vi "生成与显示信号.vi"() -> ()   [LabVIEW 2010]
doc: "Use this template to generate a signal and display the generated data in a graph. \n\nUse this template with the exercises in the Getting Started with LabVIEW manual.\n\nNote: VIs created from this template will have automatic error handling enabled by default."
uses:
  Instance           1 22Saved   生成与显示信号 .vi
  Instance           2 22Saved   生成与显示信号 .vi
panel:
  out "最小值":dbl
  out "最大值":dbl
  out "算术平均值":dbl
  in  "噪声幅度":dbl(slide) scale=0.0..10.0
  out "Waveform Graph":dynamicdata(graph)
  in  "stop":bool
  # "生成与显示信号"
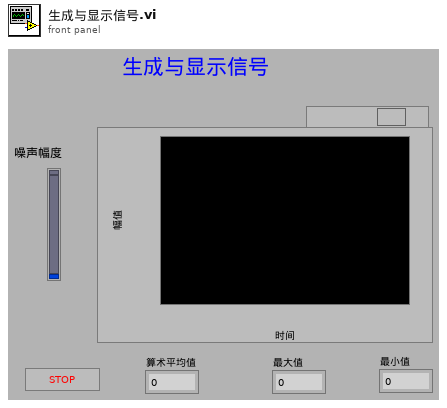
[diagram p1: front panel]
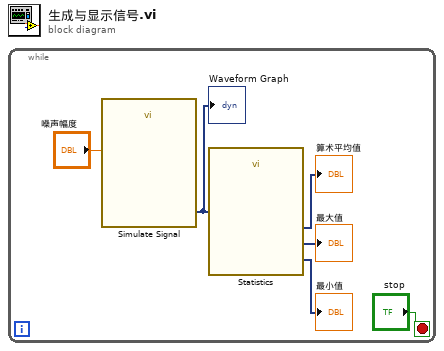
[diagram p0: block diagram]
diagram:
  n1 = while {
    stop <- "stop" stop-if-true
    n2 = call "Simulate Signal"("噪声幅值"="噪声幅度") -> ("三角与均匀噪声"=w5:dynamicdata)  [unwired: 13 in, 1 out]
    "Waveform Graph" <- w5
    n3 = call "Statistics"("Signals"=w5) -> ("Arithmetic Mean"=→"算术平均值":dynamicdata, "Minimum"=→"最小值":dynamicdata, "Maximum"=→"最大值":dynamicdata)  [unwired: 23 in, 1 out]
  }
